vi "ManageQMess.vi"(8 "ErrorIn(No Error)":errorcluster caption="entrée d'erreur (pas d'erreur)", 10 "Message":string, 11 "KlingerMotor.lvclass":refnum<class "KlingerMotor.lvclass">) -> (0 "sortie d'erreur":errorcluster, 3 "KlingerMotor.lvclass Out":refnum<class "KlingerMotor.lvclass">)   [LabVIEW 2019, in "KlingerMotor.lvclass"]
uses:
  KlingerMotor.lvclass
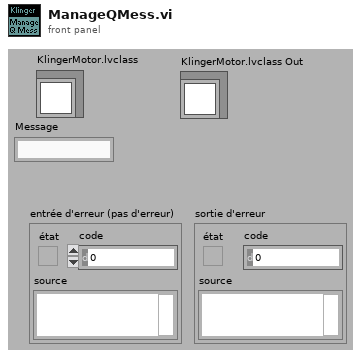
[diagram p1: front panel]
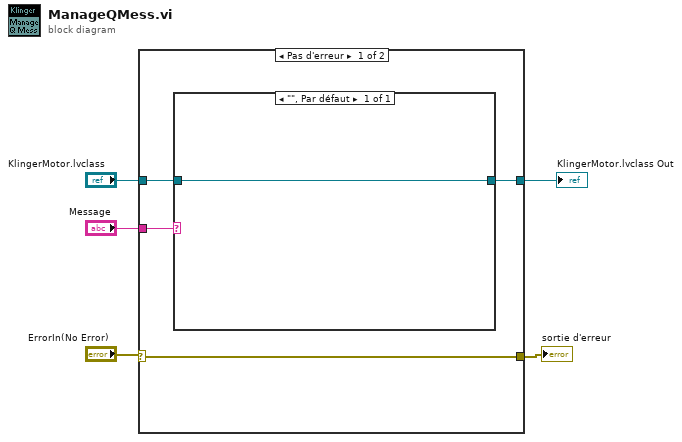
[diagram p0: block diagram]
diagram:
  n1 = case shown="Pas d'erreur" "ErrorIn(No Error)" {
    selector: "ErrorIn(No Error)" -> [w9 w12]
    tunnel: [w9 w12] -> w4
    tunnel: "Message" -> [w8 _]
    tunnel: [w7 w11] -> w2
    tunnel: "KlingerMotor.lvclass" -> [w6 w11]
    frame No Error {
      n2 = case shown="\"\", Par défaut" w8 {
        tunnel: [w10] -> w7
        tunnel: w6 -> [w10]
        frame "", Default {
        }
      }
    }
    frame Error {
    }
  }
  "sortie d'erreur" <- w4
  "KlingerMotor.lvclass Out" <- w2
